vi "Calc_rhoplus.vi"(10 "Q":dbl[](array[numeric]), 11 "P":dbl[](array[numeric])) -> (3 "rho+":dbl[](array[numeric]))   [LabVIEW 2018]
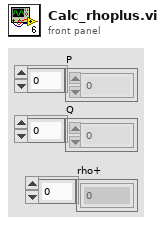
[diagram p1: front panel]
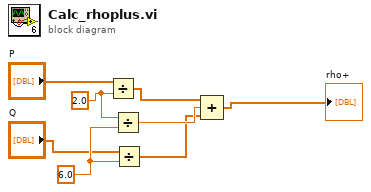
[diagram p0: block diagram]
diagram:
  w6 = 6.0
  w7 = 2.0
  n1 = Divide(x="P", y=w7) -> (x/y=w2:dbl[])
  n2 = Divide(x=w7, y=w6) -> (x/y=w4:dbl)
  n3 = Divide(x="Q", y=w6) -> (x/y=w3:dbl[])
  n4 = Compound Arithmetic op=ADD(w2, w4, w3) -> (→"rho+":dbl[])
